vi "Test Test Case Assetion Results Appended When Collecting Method Result.vi"(8 "error in (no error)":errorcluster, 11 "Test Case In":refnum<class "Result Collector Tests.lvclass">) -> (0 "error out":errorcluster, 3 "Test Case Out":refnum<class "Result Collector Tests.lvclass">)   [LabVIEW 2020, in "Result Collector Tests.lvclass"]
uses:
  Result Collector Tests.lvclass
  C:/Program Files (x86)/National Instruments/LabVIEW 2020/vi.lib/Astemes/LUnit/Test Case.lvclass
  Framework/Result Collector/Result Collector.lvclass
  Result/Result.ctl
  Result/Status.ctl
  Result/Type.ctl
  Framework/Result Collector/Result Collector.lvclass/Result Collector.ctl
  <vilib>/Astemes/LUnit/Test Case.lvclass/Test Case.ctl
  7d523b10-b8d1-4baa-9334-5865d033fd32.vi
  Framework/Result Collector/Public/API/Collect Method Results.vi
  <vilib>/Astemes/LUnit/Palette/Pass.vi
  <vilib>/Astemes/LUnit/Palette/Fail.vi
  <vilib>/Astemes/LUnit/Compare Variants.vi
  <vilib>/Astemes/LUnit/Describe Comparison.vi
  <vilib>/Astemes/LUnit/Set Assertion Type.vi
  <vilib>/Astemes/LUnit/Add test result.vi
  <vilib>/Astemes/LUnit/Variant to string.vi
  <vilib>/Astemes/LUnit/LUnit Record Assertion Result.vi
  <vilib>/Astemes/LUnit/LUnit Aggregate Assertion Results.vi
  <vilib>/Astemes/LUnit/Method Result/LUnit Merge Status.vi
  <vilib>/Astemes/LUnit/LUnit Concatenate result strings.vi
  <vilib>/Utility/Data Type/Get Type Information.vi
  <vilib>/Utility/LVClass/Get LV Class Name.vi
  Result/Result.lvlib
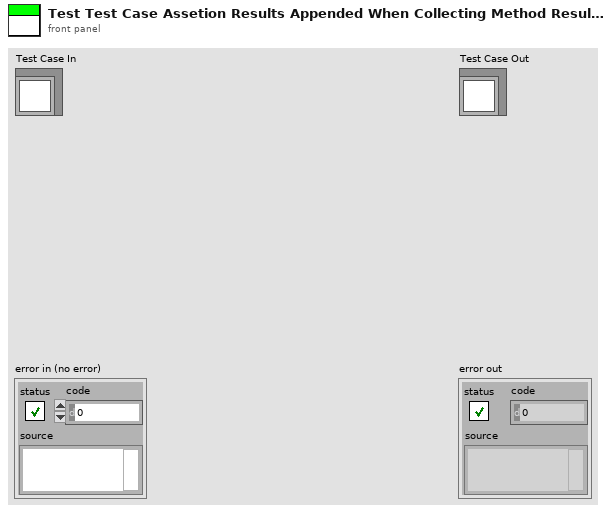
[diagram p1: front panel]
types:
  T1 = typedef "Result.lvlib/Result.ctl" = cluster{"Case":string, "Method":string, "Message":string, "Description":string, "Status":T2, "Result Type":T3}
  T2 = typedef "Result.lvlib/Status.ctl" = enum16{"Pass", "Fail", "Error", "Skipped", "Setup Error", "Broken", "Teardown Error"}
  T3 = typedef "Result.lvlib/Type.ctl" = enum16{"Assertion", "Method", "Case", "Suite"}
  T4 = typedef "Assertion Result.lvlib/Assertion Result.ctl" = cluster{"Status":T5, "Message":string, "Description":string}
  T5 = typedef "Assertion Result.lvlib/Status.ctl" = enum16{"Pass", "Fail", "Error", "Skipped", "Setup Error", "Broken", "Teardown Error"}
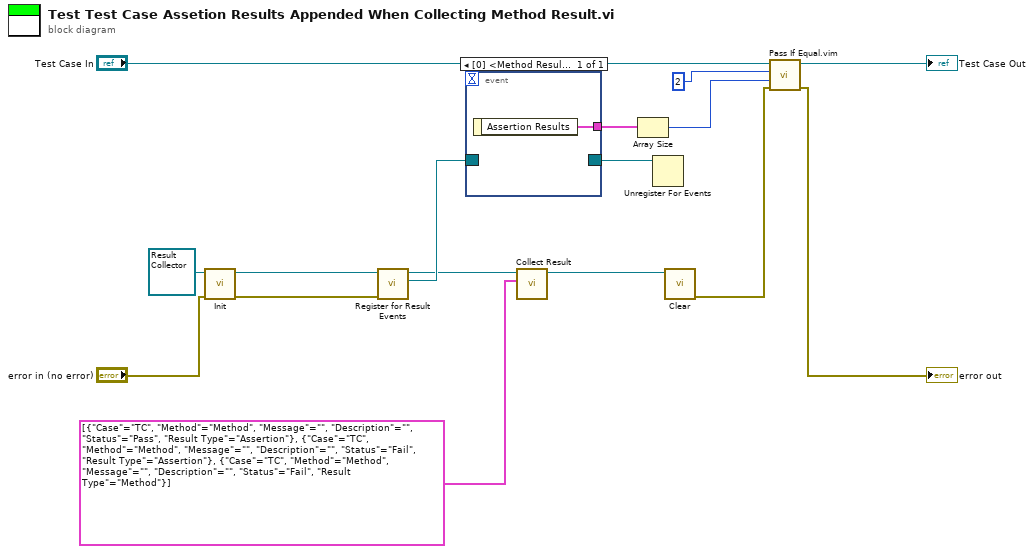
[diagram p0: block diagram]
diagram:
  n1 = call-dynamic "Init.vi"("error in (no error)"="error in (no error)", "Report Generator In"=refnum<class "Result Collector.lvclass"> refnum) -> ("error out"=w12:errorcluster, "Report Generator Out"=w13:refnum<class "Result Collector.lvclass">)  [unwired: 8 in]
  n2 = call "Register for Result Events.vi"("error in (no error)"=w12, "Result Collector In"=w13) -> ("Result Events"=w10:refnum<event-registration>, "Result Collector Out"=w8:refnum<class "Result Collector.lvclass">)  [unwired: 7 in, 1 out]
  n3 = event shown="[0] <Method Result>: User Event" {
    selector: w10 -> [_]
    dyn-events: [_] -> w9
    timeout: _ -> [_]
    tunnel: [w17] -> w5
    event User Event {
      n4 = event-data() -> ("Assertion Results"=w17:T4[])  [unwired: 1 in]
    }
  }
  n5 = call "Collect Result.vi"("Results"=T1[] [{"Case"="TC", "Method"="Method", "Message"="", "Description"="", "Status"=enum."Pass", "Result Type"=enum."Assertion"}, {"Case"="TC", "Method"="Method", "Message"="", "Description"="", "Status"=enum."Fail", "Result Type"=enum."Assertion"}, {"Case"="TC", "Method"="Method", "Message"="", "Description"="", "Status"=enum."Fail", "Result Type"=enum."Method"}], "Report Generator In"=w8) -> ("Report Generator Out"=w7:refnum<class "Result Collector.lvclass">)  [unwired: 9 in]
  n6 = Array Size(array=w5) -> (size(s)=w2:i32)
  n7 = Unregister For Events(event registration refnum=w9) -> ()  [unwired: 1 in, 1 out]
  n8 = call-dynamic "Clear.vi"("Report Generator In"=w7) -> ("error out"=w4:errorcluster)  [unwired: 9 in, 1 out]
  n9 = call "Pass If Equal.vim"("error in (no error)"=w4, "Actual"=w2, "Expected"=2 ("size(s)"), "LUnit Test Case In"="Test Case In") -> ("error out"=→"error out":errorcluster, "LUnit Test Case Out"=→"Test Case Out":refnum<class "Result Collector Tests.lvclass">)  [unwired: 6 in]
